vi "MainStates_Init.vi"(8 "error in (no error)":errorcluster, 11 "reference in":refnum<class "MainStates.lvclass"> caption="This control should only be used when\na sub class is inheriting this class") -> (0 "error out":errorcluster, 3 "reference out":refnum<class "MainStates.lvclass"> caption="This indicator should only be used when\na sub class is inheriting this class")   [LabVIEW 2019, in "MainStates.lvclass"]
uses:
  MainStates.lvclass
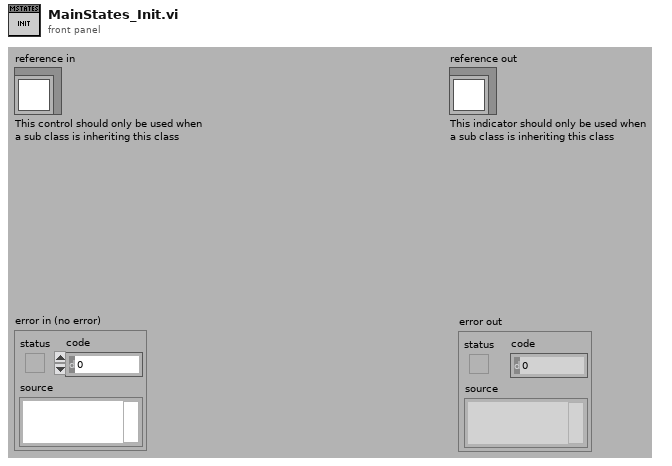
[diagram p1: front panel]
types:
  T1 = typedef "MainStates.lvclass/ObjectAttributes.ctl" = cluster{"State":T2}
  T2 = typedef "MainStates.lvclass/MainState.ctl" = enum16{"Init", "Idle", "Safe Stop", "Normal Working", "Critical Error", "Closing"}
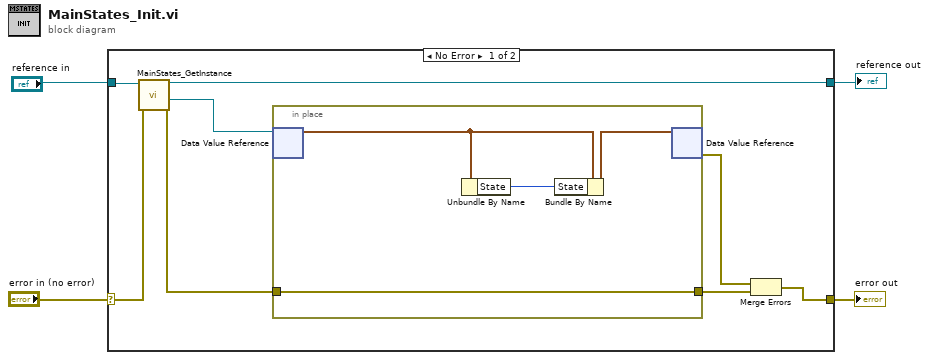
[diagram p0: block diagram]
diagram:
  n1 = case shown="No Error" "error in (no error)" {
    selector: "error in (no error)" -> [w10 w18]
    tunnel: [w11 w18] -> w3
    tunnel: "reference in" -> [w9 w17]
    tunnel: [w7 w17] -> w1
    frame No Error {
      n2 = call "MainStates_GetInstance.vi"("error in (no error)"=w10, "reference in"=w9) -> ("error out"=w6:errorcluster, "DVRRefOut"=w8:refnum<data-value>, "reference out"=w7:refnum<class "MainStates.lvclass">)  [unwired: 5 in, 2 out]
      n3 = in-place {
        in-place-border: w6 -> [w13]
        in-place-border: [w13] -> w5
        n4 = in-place-dvr #1(w8) -> (w15:T1)  [unwired: 1 out]
        n5 = Unbundle By Name(w15) -> ("State"=w14:T2)
        n6 = Bundle By Name(cluster=w15, "State"=w14) -> (w16:T1)
        n7 = in-place-dvr #1(w16) -> (w12:errorcluster)  [unwired: 1 out]
      }
      n8 = Merge Errors(w12, w5) -> (w11:errorcluster)
    }
    frame Error {
    }
  }
  "error out" <- w3
  "reference out" <- w1
